vi "DSF.Shared.Configuration.Transfer Group.Create.vi"(8 "error in (no error)":errorcluster, 11 "Transfer Group Configuration cluster":T1={"name"="", "direction"=enum."Tx", "cycle timing"={"priority"=0, "decimation"=1, "offset"=0}, "Transfers"=[], "settings"=[]}) -> (0 "error out":errorcluster, 3 "Transfer Group Configuration":refnum<class "DSF.Shared.Configuration.Transfer Group.lvclass">)   [LabVIEW 2017, in "DSF.Engine.lvlib" / "DSF.Shared.Configuration.Transfer Group.lvclass"]
uses:
  DSF.Shared.Configuration.Transfer Group.lvclass
  Typedefs/DSF Engine Transfer Group Configuration.ctl
  DSF Configuration API/1.0.0/Public/Controls/DSF Direction.ctl
  DSF Configuration API/1.0.0/Public/Controls/DSF Timing Info.ctl
  Typedefs/DSF Engine Transfer Configuration.ctl
  DSF Configuration API/1.0.0/Public/Controls/DSF Byte Order.ctl
  Typedefs/DSF Engine Channel Configuration.ctl
  DSF Configuration API/1.0.0/Public/Controls/DSF Data Type.ctl
  DSF Configuration API/1.0.0/Public/Controls/DSF Settings Info.ctl
  DSF.Shared.Configuration.Transfer Group.lvclass/DSF.Shared.Configuration.Transfer Group.ctl
  Transfer/DSF.Shared.Configuration.Transfer.lvclass
  DSF Configuration API/1.0.0/DSF Configuration API.lvlib
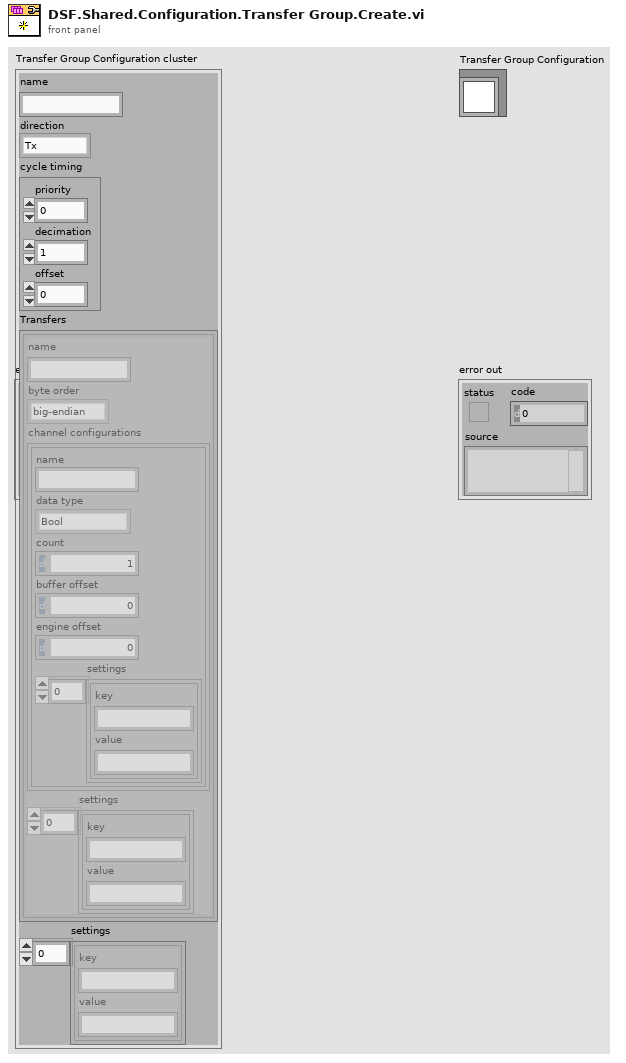
[diagram p1: front panel]
types:
  T1 = typedef "DSF Configuration API.lvlib/DSF Engine Transfer Group Configuration.ctl" = cluster{"name":string, "direction":T2, "cycle timing":T3, "Transfers":T4[], "settings":T8}
  T2 = typedef "DSF Configuration API.lvlib/DSF Direction.ctl" = enum8{"Tx", "Rx"}
  T3 = typedef "DSF Configuration API.lvlib/DSF Timing Info.ctl" = cluster{"priority":i32, "decimation":i32, "offset":i32}
  T4 = typedef "DSF Configuration API.lvlib/DSF Engine Transfer Configuration.ctl" = cluster{"name":string, "byte order":T5, "channel configurations":T6[], "settings":T8}
  T5 = typedef "DSF Configuration API.lvlib/DSF Byte Order.ctl" = enum8{"big-endian", "little-endian"}
  T6 = typedef "DSF Configuration API.lvlib/DSF Engine Channel Configuration.ctl" = cluster{"name":string, "data type":T7, "count":u64, "buffer offset":u64, "engine offset":u64, "settings":T8}
  T7 = typedef "DSF Configuration API.lvlib/DSF Data Type.ctl" = enum8{"Bool", "SGL", "DBL", "I8", "I16", "I32", "I64", "U8", "U16", "U32", "U64"}
  T8 = typedef "DSF Configuration API.lvlib/DSF Settings Info.ctl" = cluster{"key":string, "value":string}[]
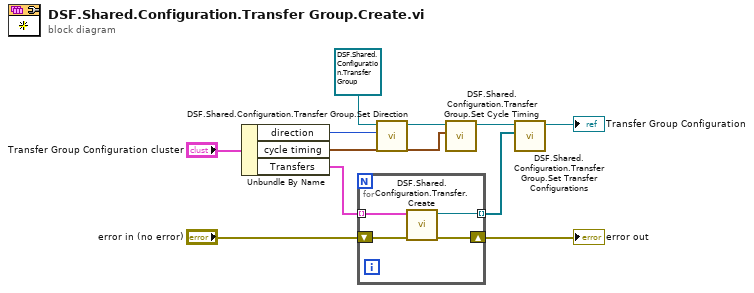
[diagram p0: block diagram]
diagram:
  n1 = Unbundle By Name("Transfer Group Configuration cluster") -> ("direction"=w5:T2, "cycle timing"=w4:T3, "Transfers"=w9:T4[])
  n2 = for {
    shift-right: [w13] -> w8
    shift-left: "error in (no error)" -> [w15]
    tunnel: w9 -> [w14] mode=indexing
    tunnel: [w12] -> w7 mode=indexing
    n3 = call "DSF.Shared.Configuration.Transfer.Create.vi"("error in (no error)"=w15, "Transfer Configuration cluster"=w14) -> ("error out"=w13:errorcluster, "Transfer Configuration out"=w12:refnum<class "DSF.Shared.Configuration.Transfer.lvclass">)  [unwired: 8 in]
  }
  "error out" <- w8
  n4 = call "DSF.Shared.Configuration.Transfer Group.Set Direction.vi"("direction"=w5, "Transfer Group Configuration in"=refnum<class "DSF.Shared.Configuration.Transfer Group.lvclass"> refnum) -> ("Transfer Group Configuration out"=w3:refnum<class "DSF.Shared.Configuration.Transfer Group.lvclass">)  [unwired: 9 in]
  n5 = call "DSF.Shared.Configuration.Transfer Group.Set Cycle Timing.vi"("cycle timing"=w4, "Transfer Group Configuration in"=w3) -> ("Transfer Group Configuration out"=w2:refnum<class "DSF.Shared.Configuration.Transfer Group.lvclass">)  [unwired: 9 in]
  n6 = call "DSF.Shared.Configuration.Transfer Group.Set Transfer Configurations.vi"("Transfer Configurations"=w7, "Transfer Group Configuration in"=w2) -> ("Transfer Group Configuration out"=→"Transfer Group Configuration":refnum<class "DSF.Shared.Configuration.Transfer Group.lvclass">)  [unwired: 9 in]
